vi "Where I Am.vi"(0 "MDF":T1) -> ()   [LabVIEW 2010]
uses:
  5.0-Global.vi
  4-High Neurons/MissionDefinitionFile.ctl
  4-High Neurons/MDFArray.ctl
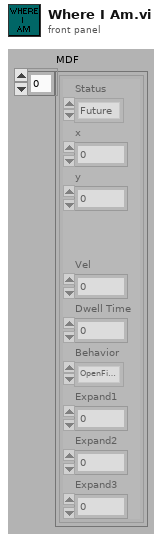
[diagram p1: front panel]
types:
  T1 = typedef "MDFArray.ctl" = T2[]
  T2 = typedef "MissionDefinitionFile.ctl" = cluster{"Status":enum16{"Past", "Current", "Future"}, "x":dbl, "y":dbl, "Vel":dbl, "Dwell Time":dbl, "Behavior":enum16{"OpenFieldTransit", "WallFollow", "LaneFollow", "ManualMode"}, "Expand1":dbl, "Expand2":dbl, "Expand3":dbl}
  T3 = cluster{"Waypoint Lat.":dbl, "Waypoint Lon.":dbl, "Current Lat.":dbl, "Current Lon. ":dbl, "Current Velocity":dbl, "Current Heading":dbl, "Desired Velocity":dbl, "Mode":enum16{"Traverse the O"}, "Status":enum16{"Current", "Future", "Past"}}[]
  T4 = cluster{"Waypoint Lat.":dbl, "Waypoint Lon.":dbl, "Current Lat.":dbl, "Current Lon. ":dbl, "Current Velocity":dbl, "Current Heading":dbl, "Desired Velocity":dbl, "Mode":enum16{"Traverse the O"}, "Status":enum16{"Current", "Future", "Past"}}
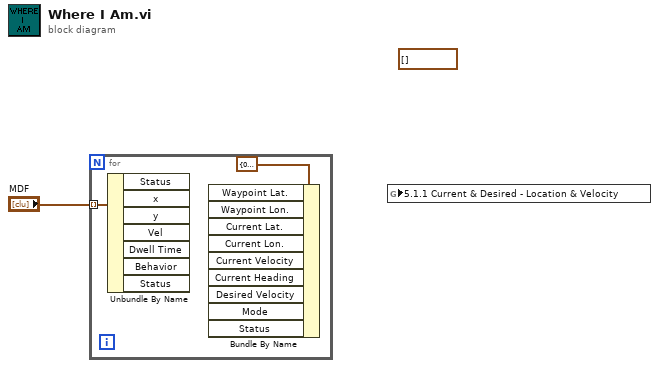
[diagram p0: block diagram]
diagram:
  (unwired) T3 [] ("5.1.1 Current & Desired - Location & Velocity")
  n1 = for {
    tunnel: "MDF" -> [w3] mode=indexing
    n2 = Unbundle By Name(w3) -> ()  [unwired: 7 out]
    n3 = Bundle By Name(cluster=T4 {"Waypoint Lat."=0.0, "Waypoint Lon."=0.0, "Current Lat."=0.0, "Current Lon. "=0.0, "Current Velocity"=0.0, "Current Heading"=0.0, "Desired Velocity"=0.0, "Mode"=enum."Traverse the O", "Status"=enum."Current"} ("Where-to-Where")) -> ()  [unwired: 9 in, 1 out]
  }
  n4 = global read "5.0-Global.vi" "5.1.1 Current & Desired - Location & Velocity"() -> ()  [unwired: 1 in]
